vi "General Config Stress Test.vi"() -> ()   [LabVIEW 2021]
uses:
  Ethernet/Config Types/General Settings.ctl
  Protocol.ctl
  Ethernet/Ethernet.lvclass
  Battery Simulator 1200 Driver.lvclass
panel:
  out "Value":string
  out "General Settings":T1
  out "Configuration Error?":bool
  out "Retrieved XML":string
  in  "stop":bool
  out "Iteration":i32
  out "Retrieved == New?":bool
  out "error out":errorcluster
  in  "UDP port":u16=54321
  in  "TCP port":u16=12345
  in  "Box IP address":string="192.168.1.100"
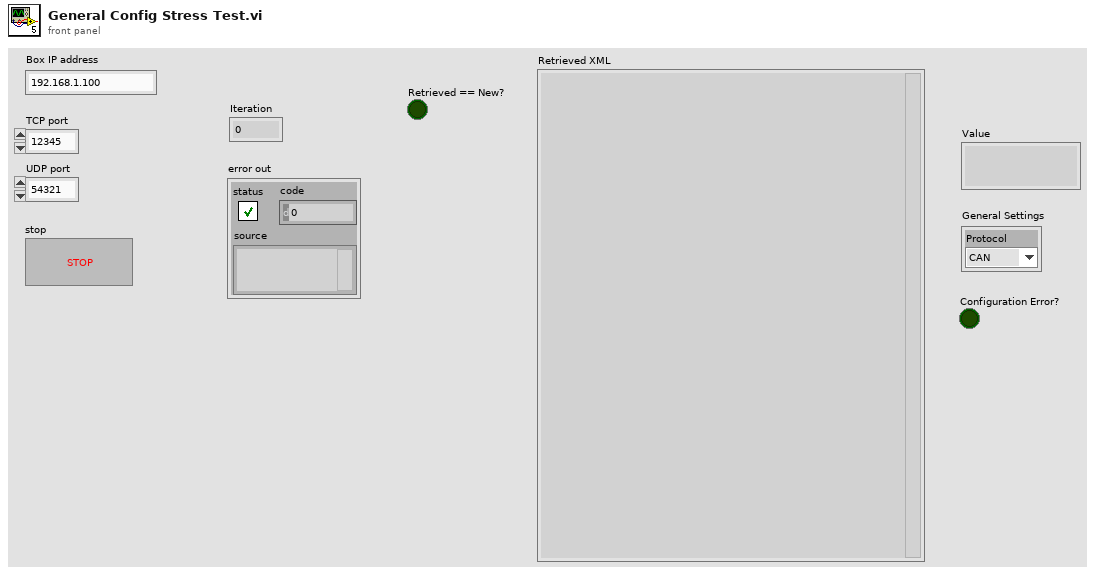
[diagram p1: front panel]
types:
  T1 = typedef "Battery Simulator 1200 LabVIEW Driver.lvlib/Ethernet.lvclass/General Settings.ctl" = cluster{"Protocol":T2}
  T2 = typedef "Battery Simulator 1200 LabVIEW Driver.lvlib/Battery Simulator 1200 Driver.lvclass/Protocol.ctl" = enum16{"CAN", "Ethernet"}
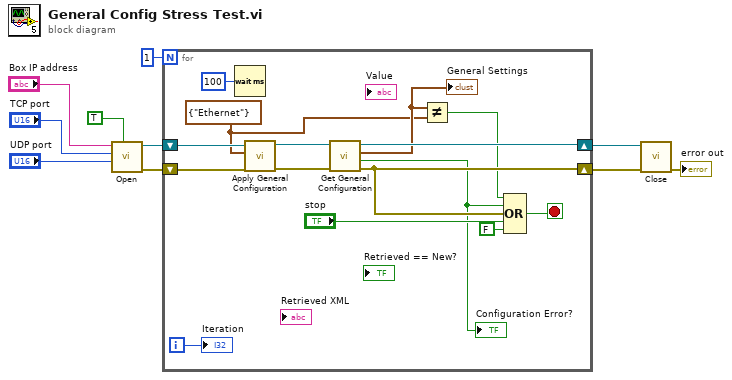
[diagram p0: block diagram]
diagram:
  n1 = call "Open.vi"("Connect for Config Only? (F)"=TRUE, "UDP port"="UDP port", "TCP port"="TCP port", "Box IP address"="Box IP address") -> ("error out"=w6:errorcluster, "ENET out"=w5:refnum<class "Ethernet.lvclass">)  [unwired: 6 in]
  n2 = for {
    N: 1 -> [_]
    shift-right: [w16] -> w4
    shift-left: w6 -> [w25]
    shift-right: [w17] -> w3
    shift-left: w5 -> [w24]
    i -> [w22]
    stop <- w21 stop-if-true
    w14 = T1 {"Protocol"=enum."Ethernet"} ("General Settings")
    n3 = Wait (ms)(milliseconds to wait=u32 100) -> ()  [unwired: 1 out]
    n4 = call "Apply General Configuration.vi"("error in (no error)"=w25, "General Settings"=w14, "Ethernet in"=w24) -> ("error out"=w19:errorcluster, "Ethernet out"=w18:refnum<class "Ethernet.lvclass">)  [unwired: 7 in]
    n5 = call "Get General Configuration.vi"("error in (no error)"=w19, "Ethernet in"=w18) -> ("error out"=w16:errorcluster, "Configuration Error?"=w12:bool, "General Settings"=w15:T1, "Ethernet out"=w17:refnum<class "Ethernet.lvclass">)  [unwired: 6 in]
    "Configuration Error?" <- w12
    "General Settings" <- w15
    n6 = Not Equal?(x=w15, y=w14) -> (x != y?=w13:bool)
    n7 = Compound Arithmetic op=OR(w13, w12, w16, "stop", FALSE ("value")) -> (w21:bool)
    "Iteration" <- w22
  }
  n8 = call-dynamic "Close.vi"("error in (no error)"=w4, "ENET in"=w3) -> ("error out"=→"error out":errorcluster)  [unwired: 9 in]
